vi "ClsNon-GeometryPeakSignal(notthicknessandpeak)IDmakerforCHRocodileII.vi"(0 "Peak Signal Name":i32(ring) items=["PeakValue", "PeakIntensity / PeakQuality", "CCDSaturation", "PeakPos", "PeakValue Median", "PeakWidth"], 1 "Peak Index":i32(ring) items=["0", "1", "2", "3", "4", "5", "6", "7", "8", "9", "10", "11", "12", "13", "14", "15"], 2 "Combination(peak or thickness)":i32(ring) items=["Peak", "Thickness"], 3 "Statistics":i32(ring) items=["Average", "Standard Deviation", "Number of valid values", "Minimum", "Maximum", "Peak-to-peak (max-min)"], 4 "Value Encoding(Nongeometric)":i32(ring) items=["For Originally Float: Float; For originally Integer: 32 bit integer", "For Originally Float: truncated 16bit integer value; For originally Integer: least significant 16 bit", "For Originally Float: 32bit integer value in 16.16 format; For originally Integer: most significant 16 bit"]) -> (5 "Non-Geometry Peak Signal ID":i32)   [LabVIEW 2010]
doc: "Non-geometric Peak Signal (not thickness and peak) ID maker(for CHRocodile 2 single/multi channel devices):\n\nGenerate the signal ID for a non-geometry peak signal(for multiple channel devices, peak signals are those appear once each channel each sample(for example, one sample in a 192-channel devices can contain only one certain global signal such as the sample counter but can contain 192 peak signals (one for each channel) such as the peak value). Geometry signals are those who should have a unit of distance. Geometry signals include distances and thickness. Non geometric peak signals are those without a distance unit, examples of which include the peak intensity/quality, the CCD position, etc..\n\nPeak Signal Name[Input]: the peak signal name.\n\nPeak Index[Input]: the index of peak of which data is acquired. $NOP will set the maximum amount of peaks available. The index of peak starts from 0.\n\nCombination[Input]: configure whether the data is a peak or a thickness(combination of two peaks).\n\nStatistics[Input]: the statistics for a given averaging period(set by AVD).\n\nValue Encoding(Nongeometric)[Input]: the encoding method for the non-geometric signals. It should be noted that for the CCD position signal, when selecting the Value Encoding as \"For Originally Float: truncated 16bit integer value; For originally Integer: least significant 16 bit\" and \"For Originally Float: 32bit integer value in 16.16 format; For originally Integer: most significant 16 bit\", the CCD position value, ,originally as a float, is multiplied by a factor of 32 before encoding in these two methods. \n\nNon-geometric peak signal ID[Output]: the calculated non-geometric peak signal ID."
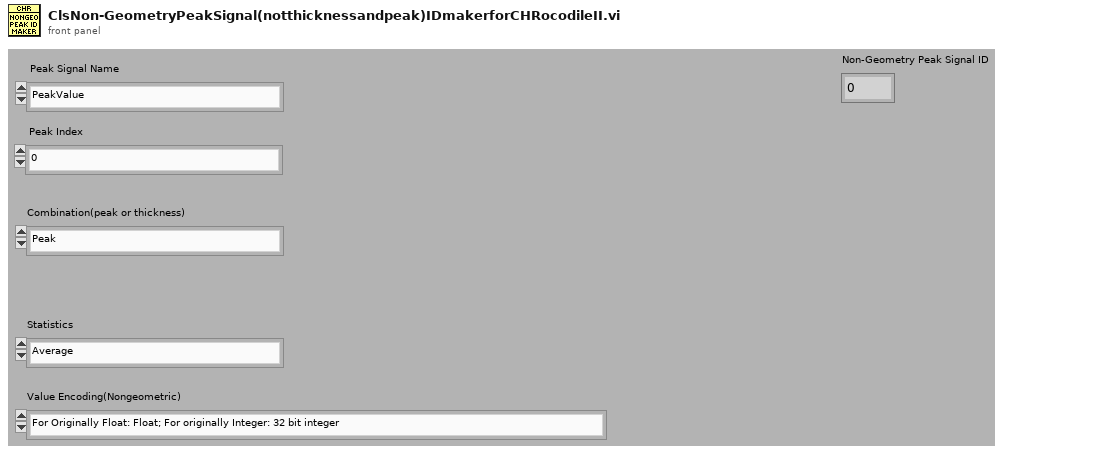
[diagram p1: front panel]
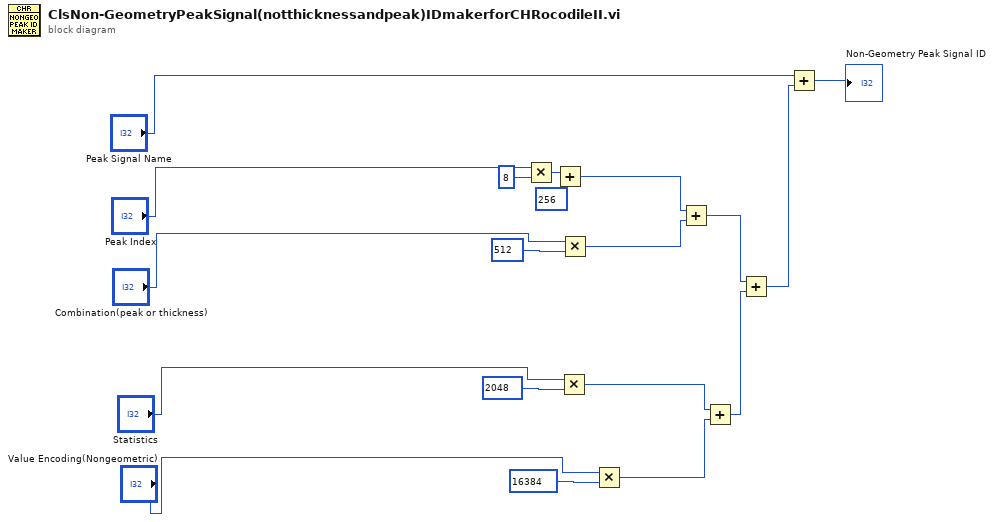
[diagram p0: block diagram]
diagram:
  n1 = Multiply(x="Peak Index", y=8) -> (x*y=w12:i32)
  n2 = Add(x=w12, y=256) -> (x+y=w7:i32)
  n3 = Multiply(x="Statistics", y=2048) -> (x*y=w5:i32)
  n4 = Multiply(x="Combination(peak or thickness)", y=512) -> (x*y=w6:i32)
  n5 = Multiply(x="Value Encoding(Nongeometric)", y=16384) -> (x*y=w4:i32)
  n6 = Add(x=w7, y=w6) -> (x+y=w3:i32)
  n7 = Add(x=w5, y=w4) -> (x+y=w2:i32)
  n8 = Add(x=w3, y=w2) -> (x+y=w1:i32)
  n9 = Add(x="Peak Signal Name", y=w1) -> (x+y=→"Non-Geometry Peak Signal ID":i32)
